vi "Create from Folder.vi"() -> ()   [LabVIEW 2020, in "GPackScratch.lvlib"]
uses:
  GPackScratch.lvlib
  GPack/Package Info.ctl
  GPack/PackageAbstract/PackageAbstract.lvclass
  GPack/GPack.lvlib
panel:
  out "error out":errorcluster
  out "Package Info":T1
  in  "Folder":path
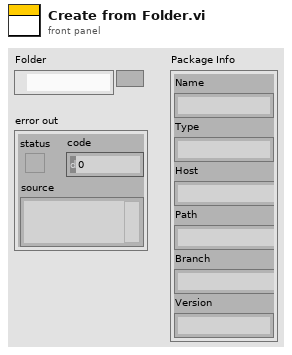
[diagram p1: front panel]
types:
  T1 = typedef "GPack.lvlib/Package Info.ctl" = cluster{"Name":string, "Type":string, "Host":string, "Path":string, "Branch":string, "Version":string}
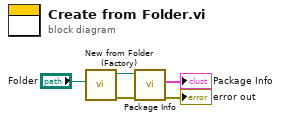
[diagram p0: block diagram]
diagram:
  n1 = call "New from Folder (Factory).vi"("Folder"="Folder") -> ("error out"=w3:errorcluster, "PackageAbstract out"=w4:refnum<class "PackageAbstract.lvclass">)  [unwired: 9 in]
  n2 = call-dynamic "Package Info.vi"("error in (no error)"=w3, "Package in"=w4) -> ("error out"=→"error out":errorcluster, "Package Info"=→"Package Info":T1)  [unwired: 7 in, 1 out]
